vi "Correction Dialogue.vi"(8 "Error In":errorcluster, 10 "Main Body Image In":T1, 11 "Provisional Line Items":T2[](array[typedef]) {"PriceIncDiscount (£)" format="%.2g"; "Discount(£)" format="%.2g"}) -> (0 "Error Out":errorcluster, 3 "ProvisionalItems":T2[](array[typedef]) {"PriceIncDiscount (£)" format="%.2g"; "Discount(£)" format="%.2g"})   [LabVIEW 2018, in "Main.lvlib"]
uses:
  Main.lvlib
  ReceiptItemInfo.ctl
  <vilib>/vision/Image Controls.llb/IMAQ Image.ctl
  <vilib>/Utility/miscctls.llb/LVPointTypeDef.ctl
  receipt parsing/Receipt Parsing.lvlib
panel:
  out "Main Body Image":T1(plugin-control)
  in  "OK Button":bool
  in  "Multicolumn Listbox":i32(listbox)
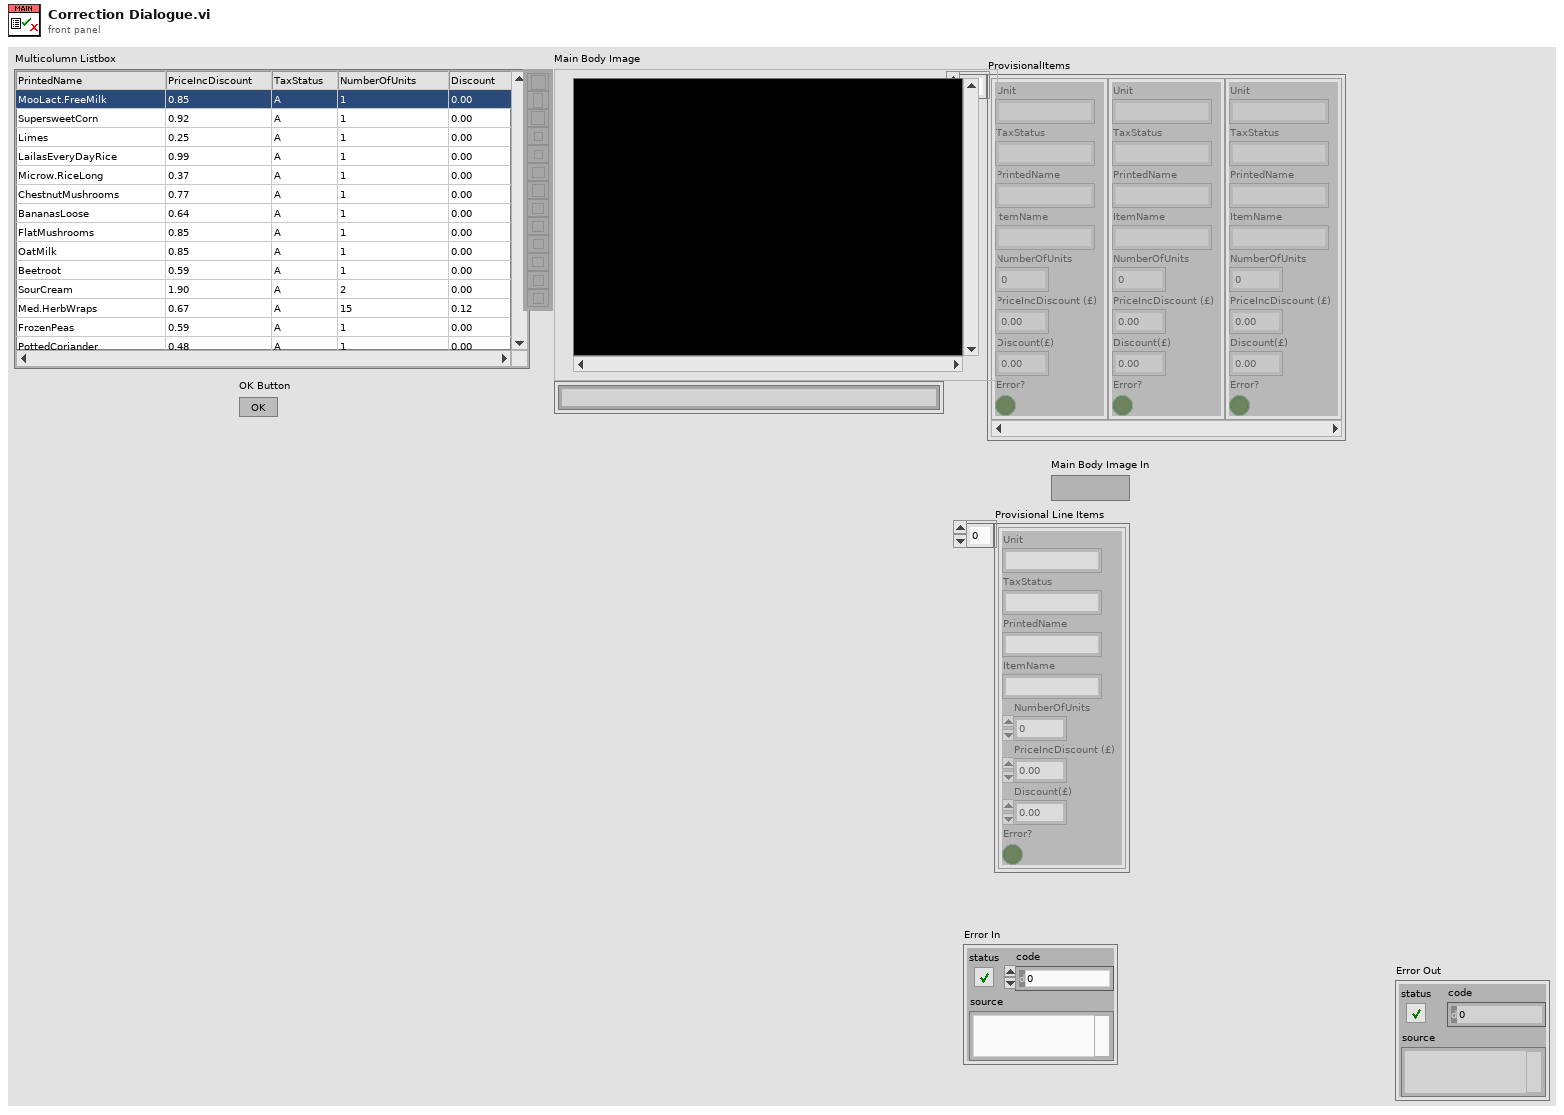
[diagram p1: front panel]
types:
  T1 = typedef "IMAQ Image.ctl" = refnum<image>
  T2 = typedef "Receipt Parsing.lvlib/ReceiptItemInfo.ctl" = cluster{"Unit":string, "TaxStatus":string, "PrintedName":string, "ItemName":string, "NumberOfUnits":dbl, "PriceIncDiscount (£)":dbl, "Discount(£)":dbl, "Error?":bool}
  T3 = typedef "LVPointTypeDef.ctl" = cluster{"Horizontal":i16, "Vertical":i16}
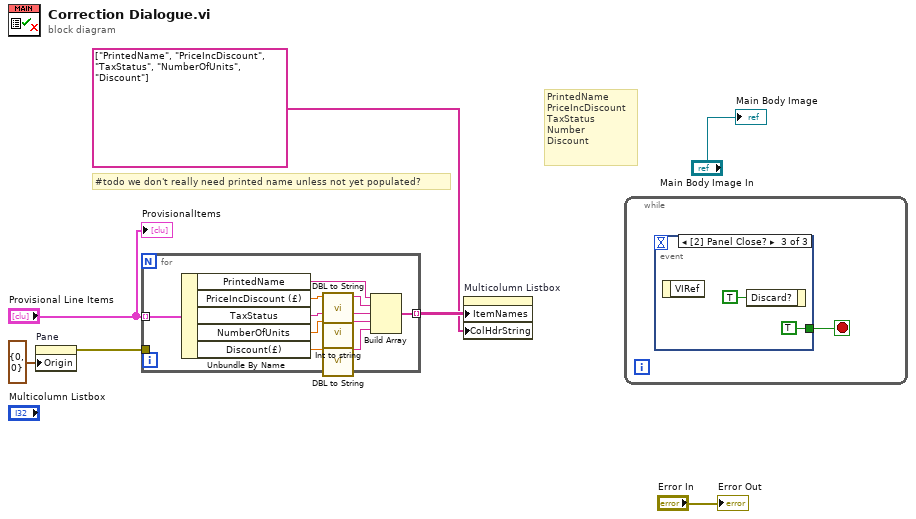
[diagram p0: block diagram]
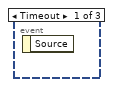
[diagram p2: hidden frame]
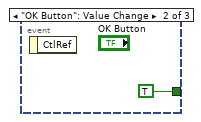
[diagram p3: hidden frame]
diagram:
  # "PrintedName\nPriceIncDiscount\nTaxStatus\nNumber\nDiscount"
  # "#todo we don't really need printed name unless not yet populated?"
  n1 = property on="Pane" class="Pane"("Origin"=T3 {"Horizontal"=0, "Vertical"=0}) -> (error out=w1:errorcluster)  [unwired: 2 in, 1 out]
  n2 = for {
    tunnel: "Provisional Line Items" -> [w17] mode=indexing
    tunnel: [w13] -> w6 mode=indexing
    tunnel: w1 -> [_]
    n3 = Unbundle By Name(w17) -> ("PrintedName"=w15:string, "PriceIncDiscount (£)"=w12:dbl, "TaxStatus"=w8:string, "NumberOfUnits"=w10:dbl, "Discount(£)"=w16:dbl)
    n4 = call "DBL to String.vi"("Number"=w12) -> ("String"=w11:string)  [unwired: 10 in]
    n5 = call "Int to string.vi"("Number"=w10) -> ("String"=w9:string)  [unwired: 10 in]
    n6 = call "DBL to String.vi"("Number"=w16) -> ("String"=w14:string)  [unwired: 10 in]
    n7 = Build Array(w15, w11, w8, w9, w14) -> (w13:string[])
  }
  n8 = property on="Multicolumn Listbox" class="MCListbox (strict)"("ItemNames"=w6, "ColHdrString"=string[] ["PrintedName", "PriceIncDiscount", "TaxStatus", "NumberOfUnits", "Discount"] ("Row Header Strings[]")) -> ()  [unwired: 2 in, 2 out]
  n9 = while {
    stop <- w18 stop-if-true
    n10 = event shown="[2] Panel Close?" {
      selector: _ -> [_ _ _]
      dyn-events: _ -> [_ _ _]
      timeout: _ -> [_ _ _]
      tunnel: [_ TRUE TRUE] -> w18
      event Timeout {
        n11 = event-data() -> ()  [unwired: 1 in, 1 out]
      }
      event "OK Button": Value Change {
        n12 = event-data() -> ()  [unwired: 1 in, 1 out]
      }
      event Panel Close? {
        n13 = event-data() -> ()  [unwired: 1 in, 1 out]
        n14 = event-data("Discard?"=TRUE) -> ()  [unwired: 1 in, 1 out]
      }
    }
  }
  "ProvisionalItems" <- "Provisional Line Items"
  "Main Body Image" <- "Main Body Image In"
  "Error Out" <- "Error In"
